vi "AlliGator Get Gated Dataset Loading Options.vi"(8 "error in (no error)":errorcluster, 11 "Image Type":string="Image") -> (0 "error out":errorcluster, 1 "Dataset Loading Options string":string, 3 "Dataset Loading Options":T1={"Pixel Well Capacity"=0, "Pile-up Correction"=FALSE, "Gate Step"=0, "Image Smoothing Options"={"Use Image Smoothing"=FALSE, "Kernel Type"=enum."Bilinear", "Bin"=1, "Algorithm"=enum."Rapid"}, "Gates to Skip"={"Start"=0, "End"=0}, "File Background Subtraction"=FALSE, "Background File Path"=path "", "Image Binning Options"={"Use Image Binning"=FALSE, "X Bin"=1, "Y Bin"=1}, "# Gates"=0, "Gates to Keep"={"First"=0, "Last"=0}, "Define Gates to"=FALSE, "Hot Pixel Removal"={"Remove Screamers"=FALSE, "Delta"=0.0, "Equalize Histogram"=FALSE, "Percentile"=0.0, "Hot Pixel Mask Image"=path "", "Use Hot Pixel Mask"=FALSE}, "Dataset Scaling Factor"=0.0, "Image Pre-processing Steps"=[]} {"Hot Pixel Removal"."Percentile" min=0 max=100; "Image Binning Options"."Y Bin" min=1; "Image Binning Options"."X Bin" min=1; "Image Smoothing Options"."Bin" min=1}, 4 "Time (s)":dbl)   [LabVIEW 2021, in "AlliGator Files.lvlib"]
doc: "Gets dataset loading options (structure + string) from stored settings."
uses:
  AlliGator Files.lvlib
  Source Image/AlliGator Image Loading Options.ctl
  Settings/AlliGator Image Smoothing Options.ctl
  Arrays/Kernel Type.ctl
  Arrays/Smoothing Algorithm.ctl
  Settings/AlliGator Background Subtraction Parameters.ctl
  Source Image/AlliGator Image Binning Options.ctl
  Settings/AlliGator Gates to Keep.ctl
  SwissSPAD/SwissSPAD Live_Image Display Options.ctl
  AlliGator Image Pre-processing Step.ctl
  Settings/AlliGator Settings List.ctl
  Decay Analysis/Decay Preprocessing/AlliGator Baseline Subtraction Method.ctl
  Settings/AlliGator Define Gates to.ctl
  Variant/Variant to Data/Variant to U32.vi
  Variant/Variant to Data/Variant to I32.vi
  Variant/Variant to Data/Variant to Boolean.vi
  Variant/Variant to Data/Variant to Path.vi
  Variant/Variant to Data/Variant to DBL.vi
  Variant/Variant to Data/Variant to [String].vi
  Settings/AlliGator Settings.lvlib
  Variant/Variant to Data/Variant to Data.lvlib
  Arrays/Arrays.lvlib
  Source Image/AlliGator Source Image.lvlib
  Decay Analysis/Decay Preprocessing/AlliGator Decay Preprocessing.lvlib
  Time/Time.lvlib
  SwissSPAD/SwissSPAD Live.lvlib
panel:
  # "see the AlliGator License on the block diagram (Ctrl+E or Window:Show Block Diagram)"
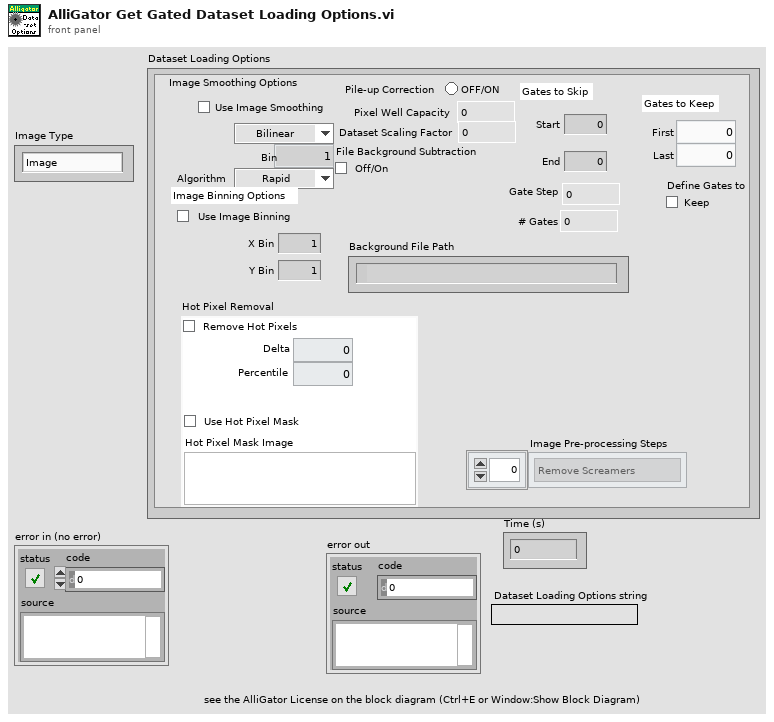
[diagram p1: front panel]
types:
  T1 = typedef "AlliGator Source Image.lvlib/AlliGator Image Loading Options.ctl" = cluster{"Pixel Well Capacity":u32, "Pile-up Correction":bool, "Gate Step":i32, "Image Smoothing Options":T2, "Gates to Skip":T5, "File Background Subtraction":bool, "Background File Path":path, "Image Binning Options":T6, "# Gates":u32, "Gates to Keep":T7, "Define Gates to":bool, "Hot Pixel Removal":T8, "Dataset Scaling Factor":dbl, "Image Pre-processing Steps":T9[]}
  T2 = typedef "AlliGator Settings.lvlib/AlliGator Image Smoothing Options.ctl" = cluster{"Use Image Smoothing":bool, "Kernel Type":T3, "Bin":i32, "Algorithm":T4}
  T3 = typedef "Arrays.lvlib/Kernel Type.ctl" = enum16{"Uniform", "Bilinear", "Gaussian"}
  T4 = typedef "Arrays.lvlib/Smoothing Algorithm.ctl" = enum16{"Rapid", "Thorough"}
  T5 = typedef "AlliGator Settings.lvlib/AlliGator Background Subtraction Parameters.ctl" = cluster{"Start":u32, "End":u32}
  T6 = typedef "AlliGator Source Image.lvlib/AlliGator Image Binning Options.ctl" = cluster{"Use Image Binning":bool, "X Bin":i32, "Y Bin":i32}
  T7 = typedef "AlliGator Settings.lvlib/AlliGator Gates to Keep.ctl" = cluster{"First":u32, "Last":u32}
  T8 = typedef "SwissSPAD Live.lvlib/SwissSPAD Live_Image Display Options.ctl" = cluster{"Remove Screamers":bool, "Delta":sgl, "Equalize Histogram":bool, "Percentile":sgl, "Hot Pixel Mask Image":path, "Use Hot Pixel Mask":bool}
  T9 = typedef "AlliGator Files.lvlib/AlliGator Image Pre-processing Step.ctl" = enum16{"Remove Screamers", "Pile-up Correction", "Binning", "Smoothing", "Rescaling", "Dead Left Column Correction"}
  T10 = typedef "AlliGator Settings.lvlib/AlliGator Settings List.ctl" = enum16{"GUI:Visible Settings Tab", "GUI:Last Run Version", "Source Image:Use Image Histogram for Contrast", "Source Image:Low Count Pixels Rejection Options", "Source Image:High Count Pixels Rejection Options", "Source Image:Use Image Brightness", "Source Image:Blend Overlay with Image Background", "Source Image:Use Fixed ROI Diameter", "Source Image:ROI Diameter", "Source Image:ROI Center Color", "Source Image:Peak Threshold", "Source Image:Intensity Threshold", "Source Image:Image Binning Options", "Source Image:Image Smoothing Options", "Source Image:Image Histogram Active", "Source Image:Invert Binary Mask", "Source Image:Hot Pixel Removal", "Source Image:Overlay Analyzed ROI Center", "Source Image:Auto-Adjust Contrast", "Source Image:Histogram Lower Percentile", "Source Image:Histogram Upper Percentile", "Source Image:Save Source Image", "Source Image:Scale Bar Options", "Source Image:Image Resolution (Pixel Size)", "Source Image:Flatfield Correction", "Source Image:Show Dead Left Columns Correction", "Source Image:Dead Left Columns Correction", "Source Image:Image Pre-Processing Operations Order", "Source Image:Overlay ROI Median", "Source Image:Median Overlay Color", "Data Information:Gate Width", "Data Information:Nanotime Gate Separation", "Data Information:Macrotime Gate Separation", "Data Information:Gate Step", "Data Information:# Gates", "Data Information:Gate Image Exposure", "Data Information:Gate Image Integration", "Data Information:Gates to Skip", "Data Information:Gates to Keep", "Data Information:Define Gates to", "Data Information:Channel Name", "Data Information:Available Channel Names", "Data Information:Channel Arithmetic", "Data Information:Background File Subtraction", "Data Information:Background File", "Data Information:Background Scaling Factor", "Data Information:Background Pile-up Correction", "Data Information:Background Pixel Well Capacity", "Data Information:Laser Period", "Data Information:SYNC Period", "Data Information:Pile-up Correction", "Data Information:Pixel Well Capacity", "Data Information:Dataset Scaling Factor", "Fluorescence Decay_Decay Pre-Processing:Reverse Gates", "Fluorescence Decay_Decay Pre-Processing:Verbose Decay Pre-Processing", "Fluorescence Decay_Decay Pre-Processing:Use Decay Pre-Processing", "Fluorescence Decay_Decay Pre-Processing:Background Subtraction", "Fluorescence Decay_Decay Pre-Processing:Background Definition Range", "Fluorescence Decay_Decay Pre-Processing:Baseline Subtraction Method", "Fluorescence Decay_Decay Pre-Processing:Decay Pre-Processing Operations Order", "Fluorescence Decay_Decay Pre-Processing:Smoothing Parameter", "Fluorescence Decay_Decay Pre-Processing:Shift Decay", "Fluorescence Decay_Decay Pre-Processing:Decay Shift Parameters", "Fluorescence Decay_Decay Pre-Processing:Fold Decay", "Fluorescence Decay_Decay Pre-Processing:# Folds", "Fluorescence Decay_Decay Pre-Processing:1-Normalize Decay", "Fluorescence Decay_Decay Pre-Processing:[0-1]-Normalize Decay", "Fluorescence Decay_Decay Pre-Processing:Smoothen Decay", "Fluorescence Decay_Decay Pre-Processing:Extrapolate Decay", "Fluorescence Decay_Decay Pre-Processing:Use Periodicity", "Fluorescence Decay_Decay Pre-Processing:Use Cursors", "Fluorescence Decay_Decay Pre-Processing:Tail Fraction", "Fluorescence Decay_Decay Pre-Processing:Head Fraction", "Fluorescence Decay_Decay Pre-Processing:Additional Points", "Fluorescence Decay_Decay Pre-Processing:Straighten Decay", "Fluorescence Decay_Decay Pre-Processing:Constant Background", "Fluorescence Decay_Decay Pre-Processing:Pixel-Normalize Decay", "Fluorescence Decay_Advanced Analysis:Extract IRF instead of Decay", "Fluorescence Decay_Advanced Analysis:IRF Extraction Options", "Fluorescence Decay_Advanced Analysis:IRF Optimization Options", "Fluorescence Decay_Advanced Analysis:Square Pulse Options", "Fluorescence Decay_Advanced Analysis:IRF Order", "Fluorescence Decay_Advanced Analysis:IRF Time Constants", "Fluorescence Decay_Advanced Analysis:Wavelet Analysis Options", "Fluorescence Decay_Advanced Analysis:Average Lifetime Options", "Fluorescence Decay_Fit Options:Fit Options", "Fluorescence Decay_Fit Options:Use Legacy Fitting Approach", "Fluorescence Decay_Fit Options:Use Data Information Laser Period", "Fluorescence Decay_Fit Parameters:Displayed Fit Parameters", "Fluorescence Decay_Fit Parameters:Fit Parameter Constraints", "Fluorescence Decay_Fit Parameters:Export Tabulated Results", "Fluorescence Decay_Fit Parameters:MLE Baseline Offset Type", "Fluorescence Decay_Fit Parameters:MLE Baseline Offset", "Fluorescence Decay_Fit Parameters:Guess Parameter Names", "Fluorescence Decay_Fit Parameters:Guess Parameter Values", "Fluorescence Decay_Fit Parameters:Guess Parameters Options", "Fluorescence Decay_Styles:Show Last Decay Only", "Fluorescence Decay_Styles:Decay Graph Color Array", "Fluorescence Decay:Decay Graph Active", "Fluorescence Decay Statistics:Min Peak Value", "Fluorescence Decay Statistics:Reject Low Decay Peak Pixels", "Fluorescence Decay Statistics:Reject High Decay Peak Pixels", "Fluorescence Decay Statistics:Max Peak Value", "Time Traces:Use File Timestamp", "Time Traces:Time Step", "Time Traces:Use Intensity Correction File", "Time Traces:Intensity Correction File", "Phasor Plot:Phasor Plot Smoothing Options", "Phasor Plot:Phasor Plot Size", "Phasor Plot:Phasor Plot Graphics Options", "Phasor Plot:Cumulative Phasor Plot", "Phasor Plot:Use Phasor Brightness", "Phasor Plot:Blend Overlay with Phasor Background", "Phasor Plot:Save Phasor Plot", "Phasor Plot:Show References", "Phasor Plot:Phasor Ratio Decay Range", "Phasor Plot:Exponential Fading", "Phasor Plot:Phasor Ratio Reference Colors", "Phasor Plot:Reference Radius", "Phasor Plot:Show Color Map Vertices", "Phasor Plot:Phasor Plot Active", "Phasor Plot:Phasor Ratio Color Map Type", "Phasor Plot:Phasor Ratio Color Map", "Phasor Plot:Phasor Ratio Display Range", "Phasor Plot:Selected Image ROI(s)", "Phasor Plot:All Image ROIs", "Phasor Plot:Selected Phasor Plot ROI(s)", "Phasor Plot:All Phasor Plot ROIs", "Phasor Plot:Phasor Ratio Color-Coded Quantity", "Phasor Plot:Store Phasor Harmonics", "Phasor Plot:Draw Reference Segment", "Phasor Plot:User-Defined Quantity", "Phasor Graph:Phasor Frequency", "Phasor Graph:Phasor Ratio Type", "Phasor Graph:Pixel-level Phasor Computation", "Phasor Graph:Save Phasor Graph", "Phasor Graph:Phasor Graph Active", "Phasor Graph:Phasor SDV Options", "Phasor Calibration:Use Backup Calibration if needed", "Phasor Graph:Define Shortest Lifetime as", "Phasor Calibration:Backup Calibration Type", "Phasor Calibration:Calibration Type", "Phasor Calibration:Calibration Lifetime", "Phasor Calibration:Calibration Map Algorithm", "Single-Exponential Phasor Locus (SEPL):Gate Parameters", "Single-Exponential Phasor Locus (SEPL):User-defined Gate", "Single-Exponential Phasor Locus (SEPL):User-defined IRF", "Single-Exponential Phasor Locus (SEPL):Phasor Parameters", "Single-Exponential Phasor Locus (SEPL):Decay & IRF Parameters", "Single-Exponential Phasor Locus (SEPL):Display Parameters", "Lifetime Analysis:Decay Analysis Parameters", "Lifetime Analysis:Lifetime Map Active", "Plugins:Python Settings", "Miscellaneous:Verbose Mode", "Miscellaneous:Beep after Script", "Miscellaneous:Saved Image File Format", "Miscellaneous:Exported Gate Image Settings", "Miscellaneous:Include Loading in Timing", "Miscellaneous:Verbose Settings Mode", "Miscellaneous:Histogram Options", "Miscellaneous:Beep on Error", "Miscellaneous:# Logical Processors Used", "Miscellaneous:ROI Description Max Characters", "Miscellaneous:Verbose Error Mode", "Miscellaneous:Transparent Mask Color"}
  T11 = typedef "AlliGator Settings.lvlib/AlliGator Define Gates to.ctl" = enum32{"Skip", "Keep"}
  T12 = typedef "AlliGator Decay Preprocessing.lvlib/AlliGator Baseline Subtraction Method.ctl" = enum16{"Mean", "Min", "Square Gated Single-Exponential", "File", "Constant"}
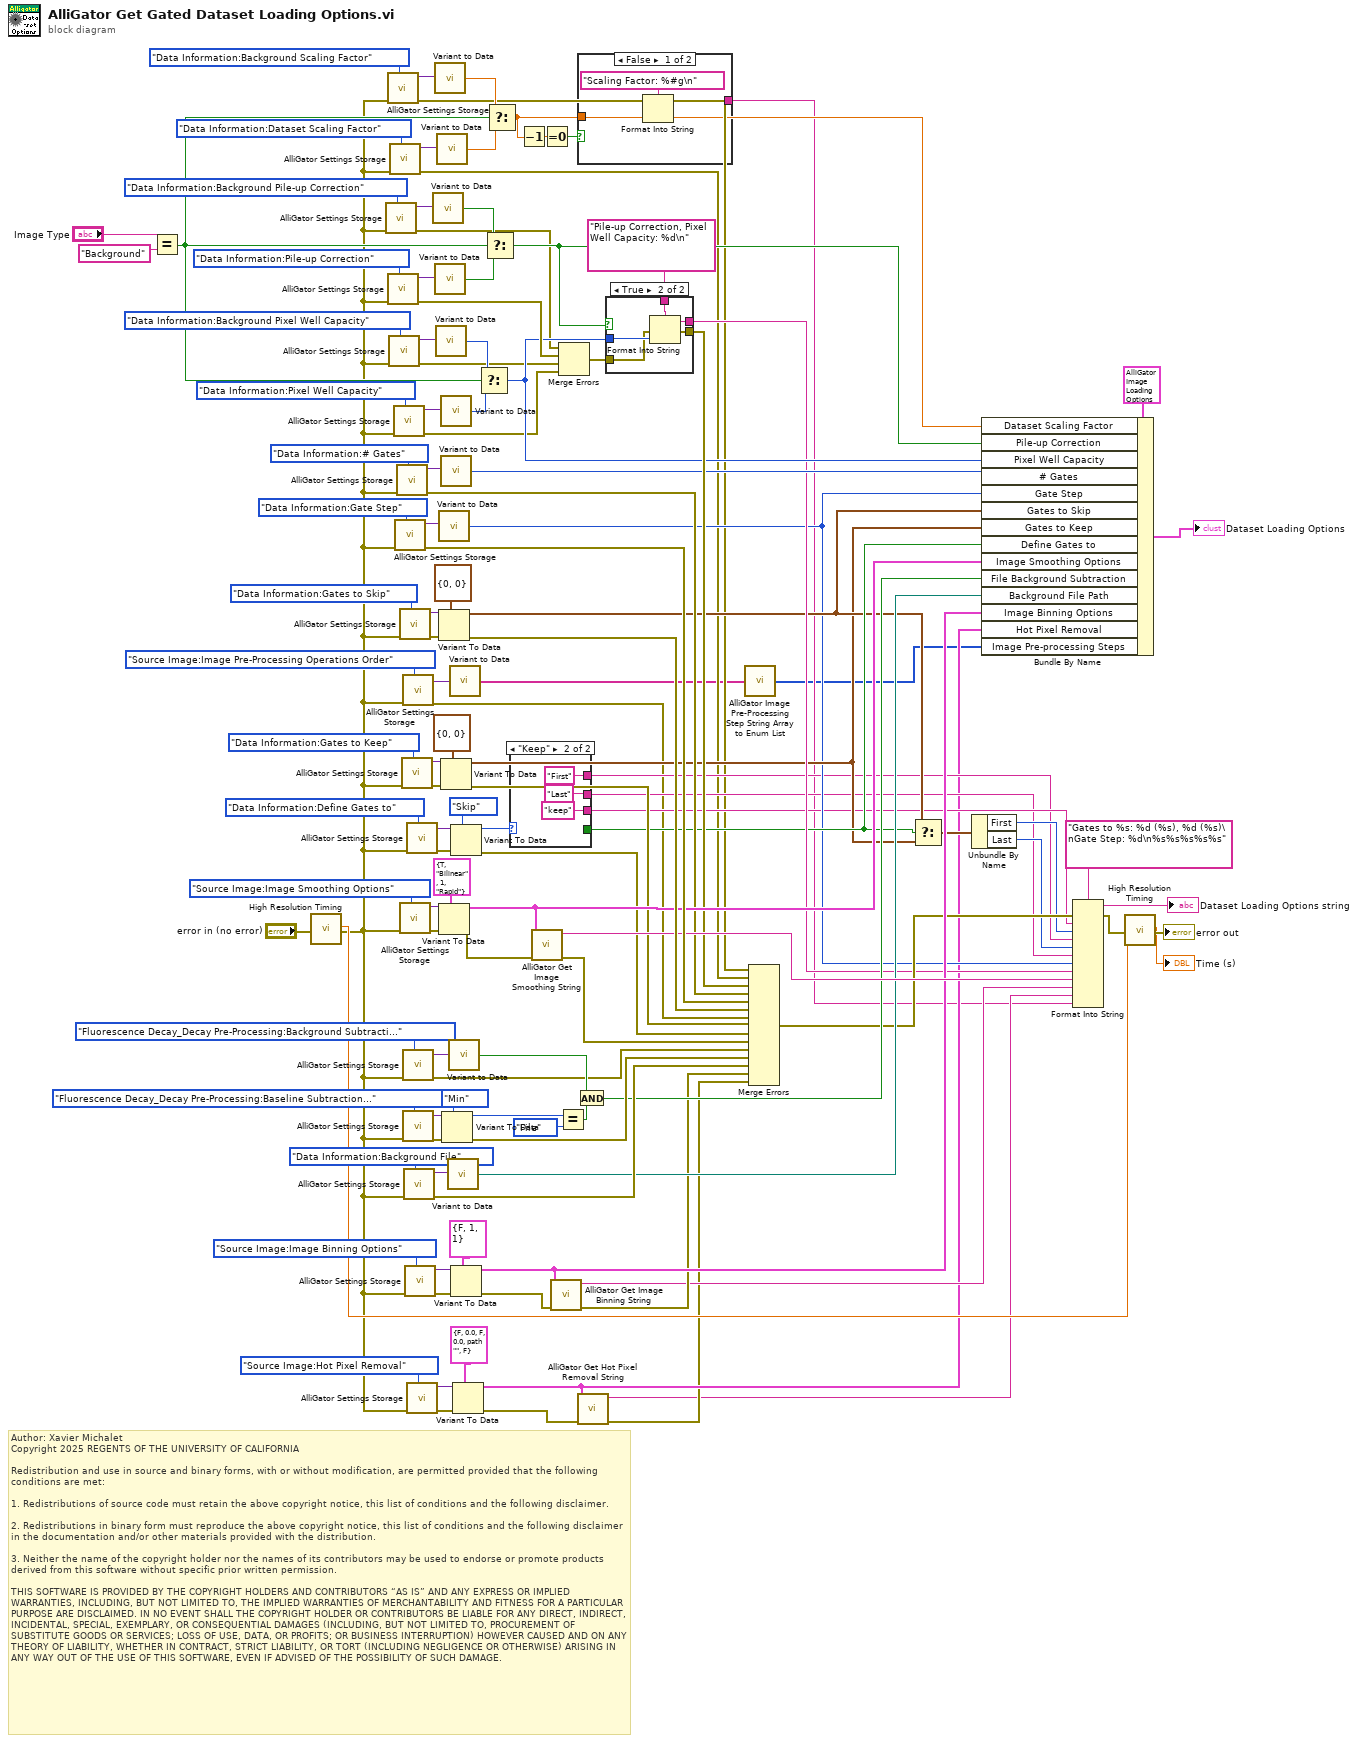
[diagram p0: block diagram]
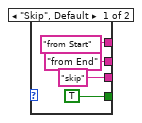
[diagram p3: hidden frame]
diagram:
  # "Author: Xavier Michalet\nCopyright 2025 REGENTS OF THE UNIVERSITY OF CALIFORNIA\n\nRedistribution and use in source and binary forms, with or without modification, are permitted provided that the following conditions are met:\n\n1. Redistributions of source code must retain the above copyright notice, this list of conditions and the following disclaimer.\n\n2. Redistributions in binary form must reproduce the above copyright notice, this list of conditions and the following disclaimer in the documentation and/or other materials provided with the distribution.\n\n3. Neither the name of the copyright holder nor the names of its contributors may be used to endorse or promote products derived from this software without specific prior written permission.\n\nTHIS SOFTWARE IS PROVIDED BY THE COPYRIGHT HOLDERS AND CONTRIBUTORS “AS IS” AND ANY EXPRESS OR IMPLIED WARRANTIES, INCLUDING, BUT NOT LIMITED TO, THE IMPLIED WARRANTIES OF MERCHANTABILITY AND FITNESS FOR A PARTICULAR PURPOSE ARE DISCLAIMED. IN NO EVENT SHALL THE COPYRIGHT HOLDER OR CONTRIBUTORS BE LIABLE FOR ANY DIRECT, INDIRECT, INCIDENTAL, SPECIAL, EXEMPLARY, OR CONSEQUENTIAL DAMAGES (INCLUDING, BUT NOT LIMITED TO, PROCUREMENT OF SUBSTITUTE GOODS OR SERVICES; LOSS OF USE, DATA, OR PROFITS; OR BUSINESS INTERRUPTION) HOWEVER CAUSED AND ON ANY THEORY OF LIABILITY, WHETHER IN CONTRACT, STRICT LIABILITY, OR TORT (INCLUDING NEGLIGENCE OR OTHERWISE) ARISING IN ANY WAY OUT OF THE USE OF THIS SOFTWARE, EVEN IF ADVISED OF THE POSSIBILITY OF SUCH DAMAGE."
  n1 = Equal?(x="Image Type", y="Background" ("x")) -> (x = y?=w15:bool)
  n2 = call "High Resolution Timing.vi"("Error In"="error in (no error)") -> ("elapsed (relative) seconds"=w29:dbl, "Error Out"=w5:errorcluster)  [unwired: 16 in, 1 out]
  n3 = call "AlliGator Settings Storage.vi"("AlliGator Settings List"=AlliGator_Settings_List."Data Information:Background Pile-up Correction", "Error In"=w5) -> ("Error Out"=w54:errorcluster, "Variant Data out"=w66:variant)  [unwired: 8 in]
  n4 = call "AlliGator Settings Storage.vi"("AlliGator Settings List"=AlliGator_Settings_List."Data Information:Background Scaling Factor", "Error In"=w5) -> ("Error Out"=w11:errorcluster, "Variant Data out"=w17:variant)  [unwired: 8 in]
  n5 = call "AlliGator Settings Storage.vi"("AlliGator Settings List"=AlliGator_Settings_List."Data Information:Pile-up Correction", "Error In"=w5) -> ("Error Out"=w74:errorcluster, "Variant Data out"=w124:variant)  [unwired: 8 in]
  n6 = call "AlliGator Settings Storage.vi"("AlliGator Settings List"=AlliGator_Settings_List."Data Information:Background Pixel Well Capacity", "Error In"=w5) -> ("Error Out"=w55:errorcluster, "Variant Data out"=w61:variant)  [unwired: 8 in]
  n7 = call "AlliGator Settings Storage.vi"("AlliGator Settings List"=AlliGator_Settings_List."Data Information:Dataset Scaling Factor", "Error In"=w5) -> ("Error Out"=w12:errorcluster, "Variant Data out"=w16:variant)  [unwired: 8 in]
  n8 = call "AlliGator Settings Storage.vi"("AlliGator Settings List"=AlliGator_Settings_List."Data Information:Pixel Well Capacity", "Error In"=w5) -> ("Error Out"=w56:errorcluster, "Variant Data out"=w125:variant)  [unwired: 8 in]
  n9 = call "AlliGator Settings Storage.vi"("AlliGator Settings List"=AlliGator_Settings_List."Data Information:Gate Step", "Error In"=w5) -> ("Error Out"=w116:errorcluster, "Variant Data out"=w123:variant)  [unwired: 8 in]
  n10 = call "AlliGator Settings Storage.vi"("AlliGator Settings List"=AlliGator_Settings_List."Data Information:# Gates", "Error In"=w5) -> ("Error Out"=w71:errorcluster, "Variant Data out"=w72:variant)  [unwired: 8 in]
  n11 = call "AlliGator Settings Storage.vi"("AlliGator Settings List"=AlliGator_Settings_List."Data Information:Gates to Skip", "Error In"=w5) -> ("Error Out"=w121:errorcluster, "Variant Data out"=w118:variant)  [unwired: 8 in]
  n12 = call "AlliGator Settings Storage.vi"("AlliGator Settings List"=AlliGator_Settings_List."Source Image:Image Smoothing Options", "Error In"=w5) -> ("Error Out"=w111:errorcluster, "Variant Data out"=w113:variant)  [unwired: 8 in]
  n13 = call "AlliGator Settings Storage.vi"("AlliGator Settings List"=AlliGator_Settings_List."Data Information:Gates to Keep", "Error In"=w5) -> ("Error Out"=w51:errorcluster, "Variant Data out"=w53:variant)  [unwired: 8 in]
  n14 = call "AlliGator Settings Storage.vi"("AlliGator Settings List"=AlliGator_Settings_List."Source Image:Image Pre-Processing Operations Order", "Error In"=w5) -> ("Error Out"=w4:errorcluster, "Variant Data out"=w3:variant)  [unwired: 8 in]
  n15 = call "AlliGator Settings Storage.vi"("AlliGator Settings List"=AlliGator_Settings_List."Fluorescence Decay_Decay Pre-Processing:Background Subtraction", "Error In"=w5) -> ("Error Out"=w92:errorcluster, "Variant Data out"=w101:variant)  [unwired: 8 in]
  n16 = call "AlliGator Settings Storage.vi"("AlliGator Settings List"=AlliGator_Settings_List."Fluorescence Decay_Decay Pre-Processing:Baseline Subtraction Method", "Error In"=w5) -> ("Error Out"=w102:errorcluster, "Variant Data out"=w100:variant)  [unwired: 8 in]
  n17 = call "AlliGator Settings Storage.vi"("AlliGator Settings List"=AlliGator_Settings_List."Data Information:Background File", "Error In"=w5) -> ("Error Out"=w90:errorcluster, "Variant Data out"=w99:variant)  [unwired: 8 in]
  n18 = call "AlliGator Settings Storage.vi"("AlliGator Settings List"=AlliGator_Settings_List."Source Image:Image Binning Options", "Error In"=w5) -> ("Error Out"=w86:errorcluster, "Variant Data out"=w87:variant)  [unwired: 8 in]
  n19 = call "AlliGator Settings Storage.vi"("AlliGator Settings List"=AlliGator_Settings_List."Data Information:Define Gates to", "Error In"=w5) -> ("Error Out"=w46:errorcluster, "Variant Data out"=w45:variant)  [unwired: 8 in]
  n20 = call "AlliGator Settings Storage.vi"("AlliGator Settings List"=AlliGator_Settings_List."Source Image:Hot Pixel Removal", "Error In"=w5) -> ("Error Out"=w24:errorcluster, "Variant Data out"=w27:variant)  [unwired: 8 in]
  n21 = call-poly "Variant to Data.vi"("Variant"=w66) -> ("Value"=w64:bool)  [unwired: 8 in]
  n22 = call-poly "Variant to Data.vi"("Variant"=w17) -> ("Value"=w18:dbl)  [unwired: 8 in]
  n23 = call-poly "Variant to Data.vi"("Variant"=w124) -> ("Value"=w63:bool)  [unwired: 8 in]
  n24 = call-poly "Variant to Data.vi"("Variant"=w61) -> ("Value"=w59:u32)  [unwired: 8 in]
  n25 = call-poly "Variant to Data.vi"("Variant"=w16) -> ("Value"=w19:dbl)  [unwired: 8 in]
  n26 = call-poly "Variant to Data.vi"("Variant"=w123) -> ("Value"=w35:i32)  [unwired: 8 in]
  n27 = Variant To Data(error in=w121, type=T5 {"Start"=0, "End"=0} ("Decay Points to Skip"), Variant=w118) -> (data=w39:T5, error out=w117:errorcluster)
  n28 = Variant To Data(error in=w111, type=T2 {"Use Image Smoothing"=TRUE, "Kernel Type"=enum."Bilinear", "Bin"=1, "Algorithm"=enum."Rapid"} ("Image Binning Options"), Variant=w113) -> (data=w80:T2, error out=w83:errorcluster)
  n29 = call-poly "Variant to Data.vi"("Variant"=w125) -> ("Value"=w58:u32)  [unwired: 8 in]
  n30 = call-poly "Variant to Data.vi"("Variant"=w72) -> ("Value"=w70:u32)  [unwired: 8 in]
  n31 = Variant To Data(error in=w51, type=T7 {"First"=0, "Last"=0} ("Decay Points to Skip"), Variant=w53) -> (data=w38:T7, error out=w49:errorcluster)
  n32 = Variant To Data(error in=w102, type=AlliGator_Baseline_Subtraction_Method."Min" ("Baseline Subtraction Method"), Variant=w100) -> (data=w95:T12, error out=w91:errorcluster)
  n33 = call-poly "Variant to Data.vi"("Variant"=w99) -> ("Path"=w88:path)  [unwired: 8 in]
  n34 = call-poly "Variant to Data.vi"("Variant"=w101) -> ("Value"=w97:bool)  [unwired: 8 in]
  n35 = call-poly "Variant to Data.vi"("Variant"=w3) -> ("String Array"=w1:string[])  [unwired: 8 in]
  n36 = Variant To Data(error in=w46, type=AlliGator_Define_Gates_to."Skip" ("Define Gates to"), Variant=w45) -> (data=w42:T11, error out=w44:errorcluster)
  n37 = Variant To Data(error in=w86, type=T6 {"Use Image Binning"=FALSE, "X Bin"=1, "Y Bin"=1} ("Image Binning Options"), Variant=w87) -> (data=w79:T6, error out=w81:errorcluster)
  n38 = Variant To Data(error in=w24, type=T8 {"Remove Screamers"=FALSE, "Delta"=0.0, "Equalize Histogram"=FALSE, "Percentile"=0.0, "Hot Pixel Mask Image"=path "", "Use Hot Pixel Mask"=FALSE} ("Hot Pixel Removal"), Variant=w27) -> (data=w23:T8, error out=w22:errorcluster)
  n39 = Select(t=w59, s=w15, f=w58) -> (s? t:f=w57:u32)
  n40 = Select(t=w64, s=w15, f=w63) -> (s? t:f=w62:bool)
  n41 = Select(t=w18, s=w15, f=w19) -> (s? t:f=w8:dbl)
  n42 = case shown="\"Keep\"" w42 {
    tunnel: [TRUE _] -> w40
    tunnel: ["skip" ("input 1") "keep" ("input 1")] -> w33
    tunnel: ["from Start" ("input 3") "First" ("input 3")] -> w32
    tunnel: ["from End" ("input 5") "Last" ("input 5")] -> w31
    frame "Skip", Default {
    }
    frame "Keep" {
    }
  }
  n43 = Decrement(x=w8) -> (x-1=w10:dbl)
  n44 = call "AlliGator Get Image Smoothing String.vi"("Error In"=w83, "Image Binning Options"=w80) -> ("Error Out"=w82:errorcluster, "String"=w105:string)  [unwired: 8 in]
  n45 = Equal To 0?(x=w10) -> (x = 0?=w9:bool)
  n46 = call "AlliGator Get Image Binning String.vi"("Error In"=w81, "Image Binning Options"=w79) -> ("Error Out"=w78:errorcluster, "String"=w77:string)  [unwired: 8 in]
  n47 = Equal?(x=w95, y=AlliGator_Baseline_Subtraction_Method."File" ("Baseline Subtraction Method")) -> (x = y?=w93:bool)
  n48 = Merge Errors(w54, w74, w55, w56) -> (w73:errorcluster)
  n49 = And(x=w97, y=w93) -> (x .and. y?=w89:bool)
  n50 = case shown="False" w9 {
    tunnel: w8 -> [w137 _]
    tunnel: [w135 _] -> w7
    frame False {
      n51 = Format Into String(format string="Scaling Factor: %#g\n", w137) -> (resulting string=w135:string)  [unwired: 2 in, 1 out]
    }
    frame True {
    }
  }
  n52 = call "AlliGator Get Hot Pixel Removal String.vi"("Error In"=w22, "Hot Pixel Removal"=w23) -> ("Error Out"=w21:errorcluster, "String"=w20:string)  [unwired: 8 in]
  n53 = case shown="True" w62 {
    tunnel: w57 -> [_ w143]
    tunnel: "Pile-up Correction, Pixel Well Capacity: %d\n" ("format string") -> [_ w142]
    tunnel: [_ w141] -> w41
    tunnel: [w138 w140] -> w76
    tunnel: w73 -> [w138 w139]
    frame False {
    }
    frame True {
      n54 = Format Into String(format string=w142, error in=w139, w143) -> (resulting string=w141:string, error out=w140:errorcluster)  [unwired: 1 in]
    }
  }
  n55 = call "AlliGator Image Pre-Processing Step String Array to Enum List.vi"("String Array"=w1) -> ("Image Pre-processing Steps"=w2:T9[])  [unwired: 8 in]
  n56 = Merge Errors(w11, w12, w76, w71, w116, w117, w4, w49, w44, w82, w92, w91, w90, w78, w21) -> (w75:errorcluster)
  n57 = Select(t=w39, s=w40, f=w38) -> (s? t:f=w37:T7)
  n58 = Unbundle By Name(w37) -> ("First"=w36:u32, "Last"=w34:u32)
  n59 = Bundle By Name(cluster=T1 {"Pixel Well Capacity"=0, "Pile-up Correction"=FALSE, "Gate Step"=0, "Image Smoothing Options"={"Use Image Smoothing"=TRUE, "Kernel Type"=enum."Bilinear", "Bin"=1, "Algorithm"=enum."Rapid"}, "Gates to Skip"={"Start"=0, "End"=0}, "File Background Subtraction"=FALSE, "Background File Path"=path "", "Image Binning Options"={"Use Image Binning"=FALSE, "X Bin"=1, "Y Bin"=1}, "# Gates"=0, "Gates to Keep"={"First"=0, "Last"=0}, "Define Gates to"=FALSE, "Hot Pixel Removal"={"Remove Screamers"=FALSE, "Delta"=0.0, "Equalize Histogram"=FALSE, "Percentile"=0.0, "Hot Pixel Mask Image"=path "", "Use Hot Pixel Mask"=FALSE}, "Dataset Scaling Factor"=0.0, "Image Pre-processing Steps"=[]} ("Image Loading Options"), "Dataset Scaling Factor"=w8, "Pile-up Correction"=w62, "Pixel Well Capacity"=w57, "# Gates"=w70, "Gate Step"=w35, "Gates to Skip"=w39, "Gates to Keep"=w38, "Define Gates to"=w40, "Image Smoothing Options"=w80, "File Background Subtraction"=w89, "Background File Path"=w88, "Image Binning Options"=w79, "Hot Pixel Removal"=w23, "Image Pre-processing Steps"=w2) -> (→"Dataset Loading Options":T1)
  n60 = Format Into String(format string="Gates to %s: %d (%s), %d (%s)\nGate Step: %d\n%s%s%s%s%s", error in=w75, w33, w36, w32, w34, w31, w35, w41, w105, w77, w20, w7) -> (resulting string=→"Dataset Loading Options string":string, error out=w114:errorcluster)  [unwired: 1 in]
  n61 = call "High Resolution Timing.vi"("relative seconds (NaN)"=w29, "Error In"=w114) -> ("elapsed (relative) seconds"=→"Time (s)":dbl, "Error Out"=→"error out":errorcluster)  [unwired: 15 in, 1 out]
